vi "编码器角度位置测量_单点_时钟滴答.vi"() -> ()   [LabVIEW 2013]
uses:
  <userlib>/ArtDAQ/_SubVI/ArtDAQ_CreateCIAngEncoderChan.vi
  <userlib>/ArtDAQ/_SubVI/ArtDAQ_Read Counter U32 1Samp.vi
panel:
  in  "Z索引相位":i32(ring)=10040 items=["A高B高"=10040, "A高B低"=10041, "A低B高"=10042, "A低B低"=10043]
  in  "解码类型":i32(ring)=10090 items=["X1"=10090, "X2"=10091, "X4"=10092, "双脉冲"=10313]
  out "数据(时钟滴答)":u32
  in  "初始角度":dbl
  in  "脉冲/转":u32=24
  in  "Z索引值":dbl
  in  "启用Z索引":bool
  in  "Stop":bool
  in  "计数器":string="Dev1/ctr0"
  out "错误输出":errorcluster
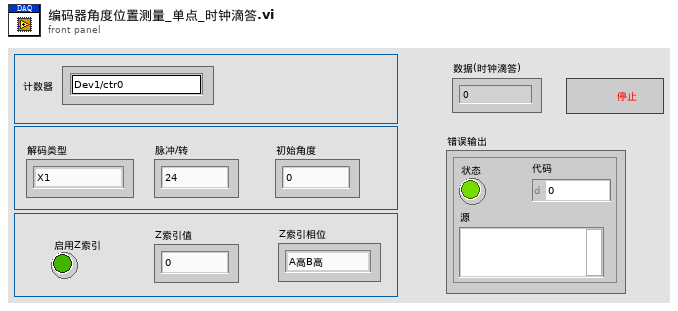
[diagram p1: front panel]
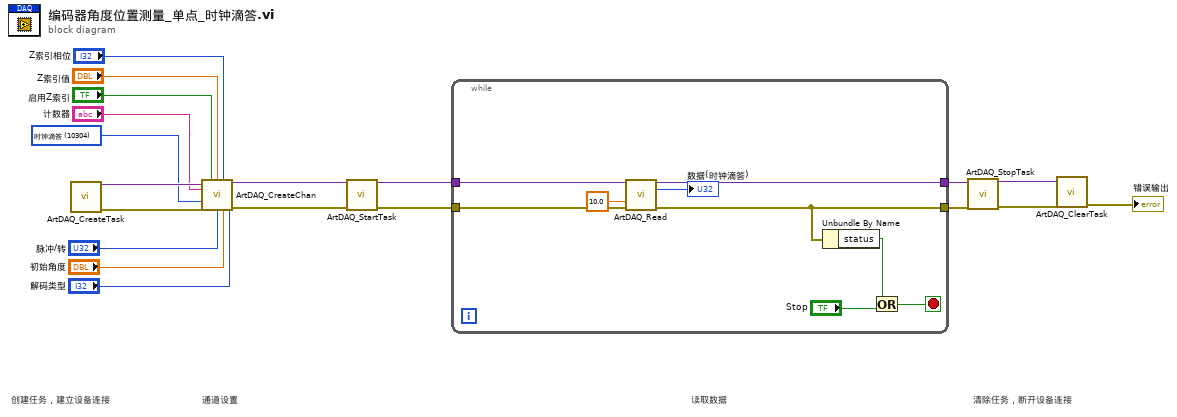
[diagram p0: block diagram]
diagram:
  w1 = 10304 items=["度"=10146, "弧度"=10273, "时钟滴答"=10304, "来自自定义换算"=10065] ("单位")
  # "清除任务，断开设备连接"
  # "读取数据"
  # "通道设置"
  # "创建任务，建立设备连接"
  n1 = call <userlib>:"ArtDAQ_CreateTask.vi"() -> ("任务句柄"=w19:variant, "错误输出"=w18:errorcluster)  [unwired: 14 in]
  n2 = call-poly <userlib>:"ArtDAQ_CreateChan.vi"("任务句柄"=w19, "启用Z索引"="启用Z索引", "Z索引值"="Z索引值", "Z索引相位"="Z索引相位", "计数器"="计数器", "解码类型"="解码类型", "单位"=w1, "错误输入"=w18, "脉冲每转"="脉冲/转", "初始角"="初始角度") -> ("任务句柄"=w5:variant, "错误输出"=w4:errorcluster)  [unwired: 4 in]
  n3 = call <userlib>:"ArtDAQ_StartTask.vi"("任务句柄"=w5, "错误输入"=w4) -> ("任务句柄"=w7:variant, "错误输出"=w6:errorcluster)  [unwired: 12 in]
  n4 = while {
    tunnel: [w28] -> w16
    tunnel: [w27] -> w14
    tunnel: w7 -> [w26]
    tunnel: w6 -> [w25]
    stop <- w22 stop-if-true
    n5 = call-poly <userlib>:"ArtDAQ_Read.vi"("任务句柄"=w26, "超时s"=10.0 ("Timeout"), "错误输入"=w25) -> ("任务句柄"=w28:variant, "数据"=→"数据(时钟滴答)":u32, "错误输出"=w27:errorcluster)  [unwired: 10 in]
    n6 = Unbundle By Name(w27) -> ("status"=w24:bool)
    n7 = Or(x=w24, y="Stop") -> (x .or. y?=w22:bool)
  }
  n8 = call <userlib>:"ArtDAQ_StopTask.vi"("任务句柄"=w16, "错误输入"=w14) -> ("任务句柄"=w15:variant, "错误输出"=w13:errorcluster)  [unwired: 12 in]
  n9 = call <userlib>:"ArtDAQ_ClearTask.vi"("任务句柄"=w15, "错误输入"=w13) -> ("错误输出"=→"错误输出":errorcluster)  [unwired: 13 in]
